vi "[Global] OperatorsImageTemplate2.vi"() -> ()   [LabVIEW 2019]
panel:
  out "OperatorsImageTemplate2Array":string[](array[string])=["OperatorsImageTemplate20", "OperatorsImageTemplate21", "OperatorsImageTemplate22", "OperatorsImageTemplate23", "OperatorsImageTemplate24", "OperatorsImageTemplate25", "OperatorsImageTemplate26", "OperatorsImageTemplate27"]
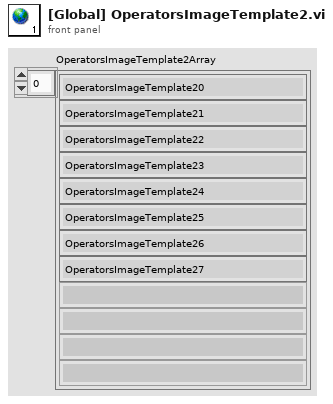
[diagram p1: front panel]
diagram:
